vi "build_data_save_paths_sysID.vi"(4 "overwrite":bool, 6 "note-blob":string, 8 "base-file-name":string="cs-traj10-500.csv", 11 "data-root":path) -> (1 "output-data-name":string, 2 "output-meta-data-path":path, 3 "output-data-path":path, 7 "input-data-path":path)   [LabVIEW 2017]
uses:
  <vilib>/regexp/Match Regular Expression.xnode
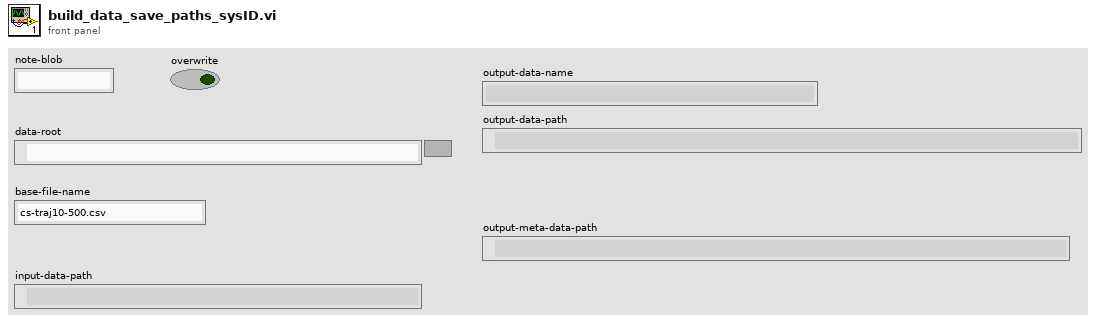
[diagram p1: front panel]
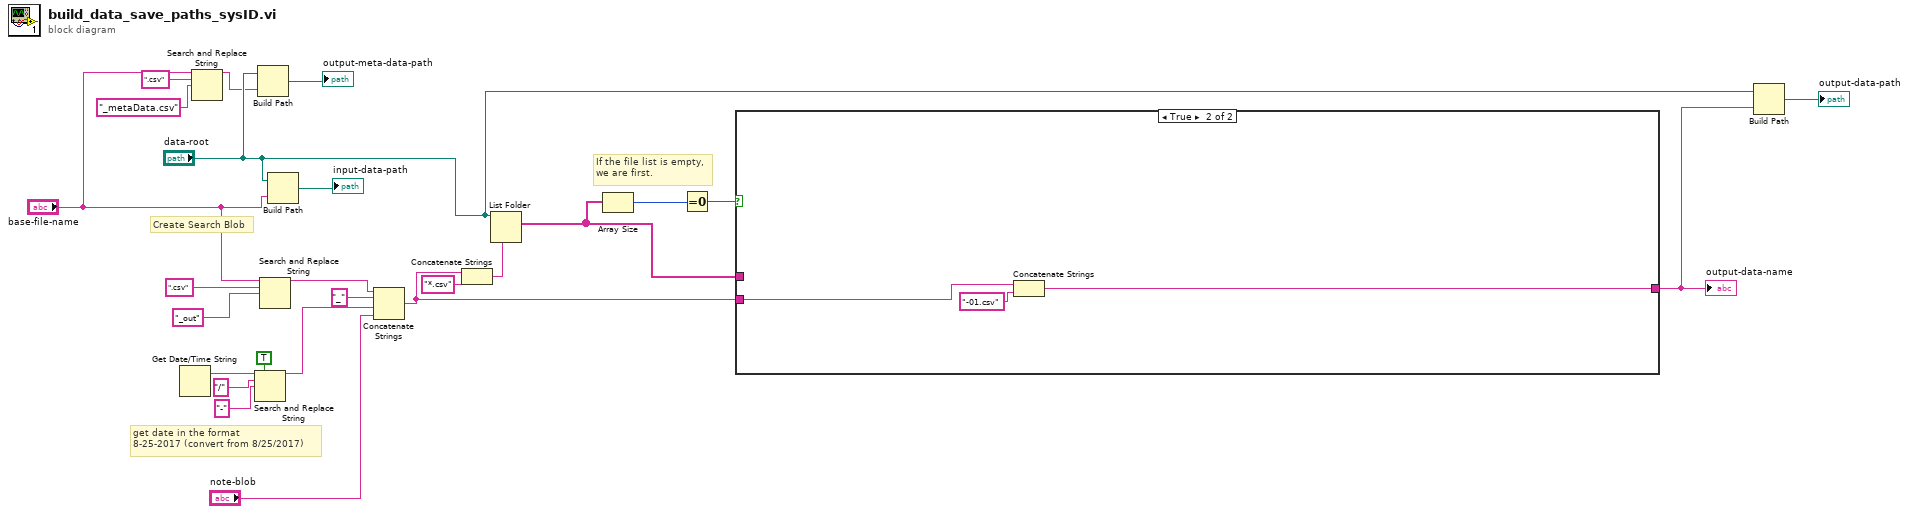
[diagram p0: block diagram]
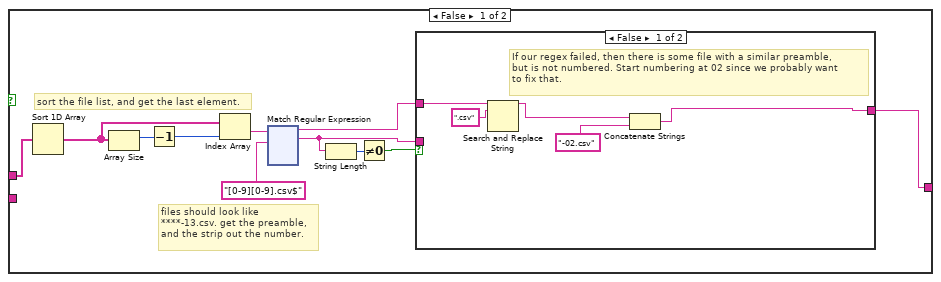
[diagram p2: hidden frame]
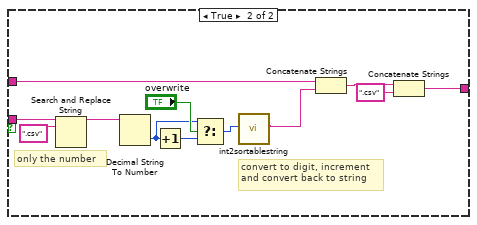
[diagram p3: hidden frame]
diagram:
  # "If the file list is empty,\nwe are first."
  # "Create Search Blob"
  # "get date in the format\n8-25-2017 (convert from 8/25/2017)"
  n1 = Get Date/Time String() -> (date string=w24:string)  [unwired: 3 in, 1 out]
  n2 = Search and Replace String(input string="base-file-name", search string=".csv", replace string="_metaData.csv" ("meta data name")) -> (result string=w1:string)  [unwired: 5 in, 3 out]
  n3 = Search and Replace String(replace all?=TRUE ("replace all? (F)"), input string=w24, search string="/", replace string="-") -> (result string=w20:string)  [unwired: 4 in, 3 out]
  n4 = Build Path(base path="data-root", name or relative path=w1) -> (appended path=→"output-meta-data-path":path)
  n5 = Search and Replace String(input string="base-file-name", search string=".csv", replace string="_out" ("replace string (\"\")")) -> (result string=w19:string)  [unwired: 5 in, 3 out]
  n6 = Build Path(base path="data-root", name or relative path="base-file-name") -> (appended path=→"input-data-path":path)
  n7 = Concatenate Strings(w19, "_", w20, "note-blob") -> (w12:string)
  n8 = Concatenate Strings(w12, "*.csv") -> (w13:string)
  n9 = List Folder(path="data-root", pattern=w13) -> (filenames=w11:string[])  [unwired: 2 in, 3 out]
  n10 = Array Size(array=w11) -> (size(s)=w16:i32)
  n11 = Equal To 0?(x=w16) -> (x = 0?=w15:bool)
  n12 = case shown="True" w15 {
    tunnel: w12 -> [_ w168]
    tunnel: [w30 w169] -> w8
    tunnel: w11 -> [w36 _]
    frame False {
      # "files should look like\n****-13.csv. get the preamble,\nand the strip out the number."
      # "sort the file list, and get the last element."
      n13 = Sort 1D Array(array=w36) -> (sorted array=w31:string[])
      n14 = Array Size(array=w31) -> (size(s)=w33:i32)
      n15 = Decrement(x=w33) -> (x-1=w32:i32)
      n16 = Index Array(array=w31, index=w32) -> (element=w35:string)
      n17 = xnode "Match Regular Expression"("input string"=w35, "regular expression"="[0-9][0-9].csv$") -> ("before match"=w29:string, "whole match"=w28:string)  [unwired: 4 in, 3 out]
      n18 = String Length(string=w28) -> (length=w27:i32)
      n19 = Not Equal To 0?(x=w27) -> (x != 0?=w26:bool)
      n20 = case shown="False" w26 {
        tunnel: w28 -> [_ w53]
        tunnel: [w41 w48] -> w30
        tunnel: w29 -> [w38 w47]
        frame False {
          # "If our regex failed, then there is some file with a similar preamble,\nbut is not numbered. Start numbering at 02 since we probably want\nto fix that."
          n21 = Search and Replace String(input string=w38, search string=".csv") -> (result string=w37:string)  [unwired: 6 in, 3 out]
          n22 = Concatenate Strings(w37, "-02.csv" ("string")) -> (w41:string)
        }
        frame True {
          # "convert to digit, increment\nand convert back to string"
          # "only the number"
          n23 = Search and Replace String(input string=w53, search string=".csv") -> (result string=w51:string)  [unwired: 6 in, 3 out]
          n24 = Decimal String To Number(string=w51) -> (number=w42:i32)  [unwired: 2 in, 1 out]
          n25 = Increment(x=w42) -> (x+1=w45:i32)
          n26 = Select(t=w42, s="overwrite", f=w45) -> (s? t:f=w44:i32)
          n27 = call "int2sortablestring.vi"("int"=w44) -> ("tens-sortable-string"=w46:string)  [unwired: 10 in]
          n28 = Concatenate Strings(w47, w46) -> (w50:string)
          n29 = Concatenate Strings(w50, ".csv" ("string")) -> (w48:string)
        }
      }
    }
    frame True {
      n30 = Concatenate Strings(w168, "-01.csv") -> (w169:string)
    }
  }
  "output-data-name" <- w8
  n31 = Build Path(base path="data-root", name or relative path=w8) -> (appended path=→"output-data-path":path)
